vi "Connect.vi"(6 "Access (R/W allowed)":T1, 7 "Mode (buffer)":u16(ring)=1 items=["commit", "buffer"], 8 "Error In":errorcluster, 11 "PVConnection in":refnum<class "PVConnection.lvclass">) -> (0 "Error Out":errorcluster, 3 "PVConnection out":refnum<class "PVConnection.lvclass">)   [LabVIEW 2014, in "CS++ProcessVariables.lvlib" / "PVConnection.lvclass"]
doc: "Open reference to a process variable."
uses:
  PVConnection.lvclass
  PVConnection.lvclass/PVConnection.ctl
  ProcessVariable/PV.lvclass/PV.ctl
  ProcessVariable/PV.lvclass
  Libraries/Utilities/CS++Utilities.lvlib
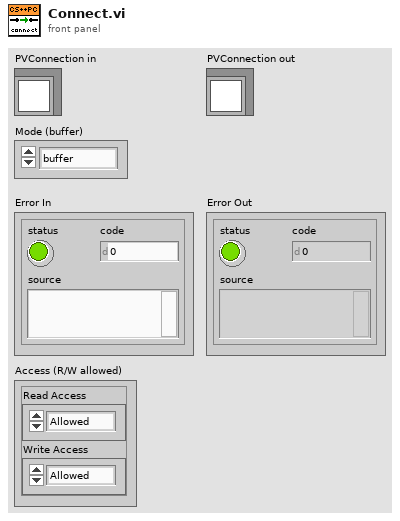
[diagram p1: front panel]
types:
  T1 = cluster{"Read Access":enum8{"Allowed", "Required", "None"}, "Write Access":enum8{"Allowed", "Required", "None"}}
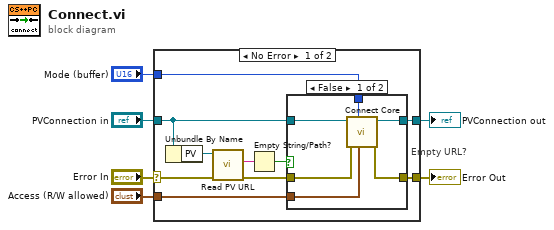
[diagram p0: block diagram]
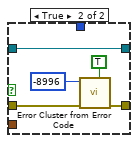
[diagram p2: hidden frame]
diagram:
  n1 = case shown="No Error" "Error In" {
    selector: "Error In" -> [w11 w29]
    tunnel: [w15 w29] -> w5
    tunnel: [w16 w28] -> w3
    tunnel: "PVConnection in" -> [w13 w28]
    tunnel: "Access (R/W allowed)" -> [w14 _]
    tunnel: "Mode (buffer)" -> [w7 _]
    frame No Error {
      n2 = Unbundle By Name(w13) -> ("PV"=w12:refnum<class "PV.lvclass">)
      n3 = call "Read PV URL.vi"("error in (no error)"=w11, "PV in"=w12) -> ("error out"=w10:errorcluster, "PV URL"=w8:string)  [unwired: 7 in, 1 out]
      n4 = Empty String/Path?(string/path=w8) -> (empty?=w9:bool)
      n5 = case "Empty URL?" shown="False" w9 {
        tunnel: [w22 w27] -> w16
        tunnel: [w21 w25] -> w15
        tunnel: w14 -> [w20 _]
        tunnel: w13 -> [w19 w27]
        tunnel: w10 -> [w18 w26]
        tunnel: w7 -> [w17 _]
        frame False {
          n6 = call-dynamic "Connect Core.vi"("Access (R/W allowed)"=w20, "Mode (commit)"=w17, "Error In"=w18, "PVConnection in"=w19) -> ("Error Out"=w21:errorcluster, "PVConnection out"=w22:refnum<class "PVConnection.lvclass">)  [unwired: 6 in]
        }
        frame True {
          n7 = call "Error Cluster from Error Code.vi"("is warning? (False)"=TRUE, "Error In"=w26, "Error Code (0)"=-8996 ("error code (no error:0)")) -> ("Error Out"=w25:errorcluster)  [unwired: 8 in]
        }
      }
    }
    frame Error {
    }
  }
  "Error Out" <- w5
  "PVConnection out" <- w3
